vi "Intan_1dstream_to_2d_samps.vi"(8 "bytes per scan":i32=72, 9 "N data scans to read":i32=1, 10 "Nchans":i32=32, 11 "1-D  data in":u16[](array[numeric])) -> (0 "Nscans read":i32, 1 "aux_cmd_array":i32[][](array[numeric]), 2 "timestamp_array":i32[](array[numeric]), 3 "2d ADCdata_array out":u16[][](array[numeric]), 4 "Nscans underflow":bool, 5 "fragmented frame read":bool)   [LabVIEW 2015]
doc: "Reformats a 1d array of U16 Intan data (written by Teensy to serial port) into a 2-D array of data.\nThis takes Nscans worth of data, each with 36 words (= 72 bytes) worth of data, and reformats into 3 arrays:\n1. 'IN' = [73, 78] ascii values from auxiliary commands (this can be checked to verify data link)\n2. 32 bit timestamp (microseconds)\n3. Nchans (=32 for now) U16s for ADC data, with data formatted as Nchans x Nsamps\n\nRead error indicators suggest possible mis-read/mis-handling of data"
panel:
  # "2-D data output"
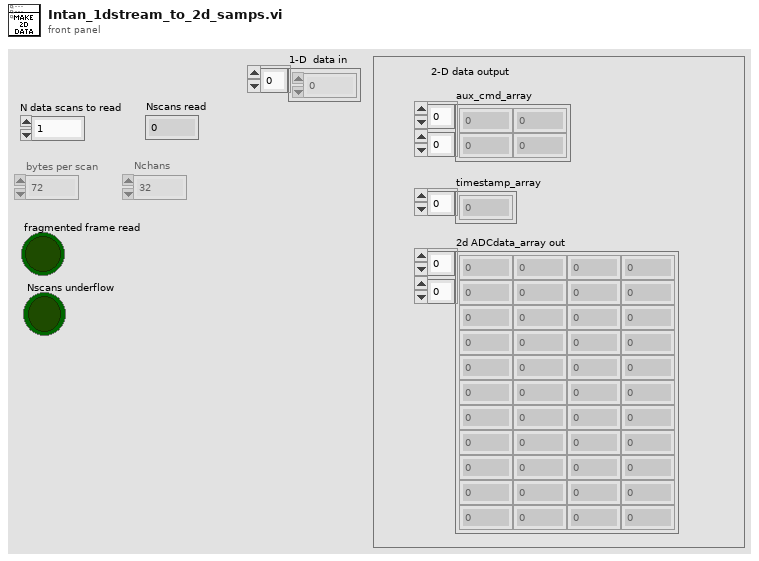
[diagram p1: front panel]
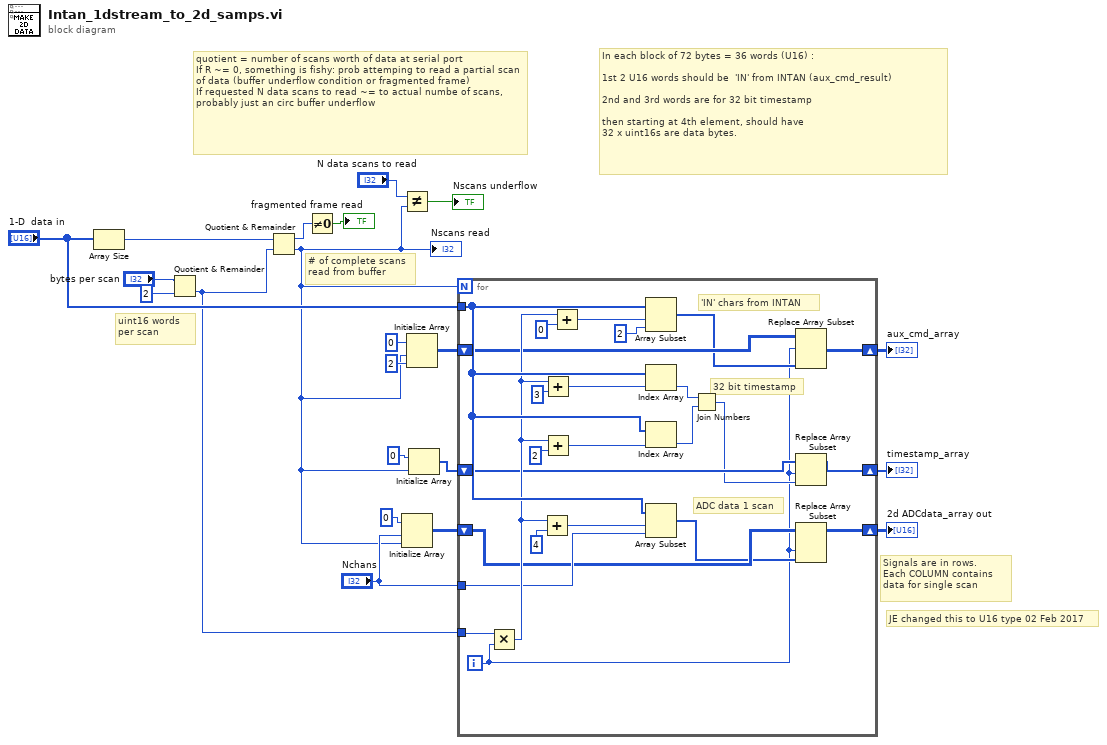
[diagram p0: block diagram]
diagram:
  # "JE changed this to U16 type 02 Feb 2017"
  # "# of complete scans\nread from buffer"
  # "Signals are in rows.\nEach COLUMN contains\ndata for single scan"
  # "In each block of 72 bytes = 36 words (U16) :\n\n1st 2 U16 words should be  'IN' from INTAN (aux_cmd_result)\n\n2nd and 3rd words are for 32 bit timestamp\n\nthen starting at 4th element, should have\n32 x uint16s are data bytes."
  # "quotient = number of scans worth of data at serial port \nIf R ~= 0, something is fishy: prob attemping to read a partial scan of data (buffer underflow condition or fragmented frame)\nIf requested N data scans to read ~= to actual numbe of scans, probably just an circ buffer underflow"
  # "uint16 words per scan"
  n1 = Array Size(array="1-D  data in") -> (size(s)=w20:i32)
  n2 = Quotient & Remainder(x="bytes per scan", y=2) -> (floor(x/y)=w15:i32)  [unwired: 1 out]
  n3 = Quotient & Remainder(x=w20, y=w15) -> (x-y*floor(x/y)=w19:i32, floor(x/y)=w1:i32)
  "Nscans read" <- w1
  n4 = Not Equal To 0?(x=w19) -> (x != 0?=→"fragmented frame read":bool)
  n5 = Not Equal?(x="N data scans to read", y=w1) -> (x != y?=→"Nscans underflow":bool)
  n6 = Initialize Array(u16 0 ("element"), "Nchans", w1) -> (w8:u16[][])
  n7 = Initialize Array(0 ("element"), w1, 2 ("dimension size")) -> (w10:i32[][])
  n8 = Initialize Array(0 ("element"), w1) -> (w9:i32[])
  n9 = for {
    N: w1 -> [_]
    tunnel: "1-D  data in" -> [w43]
    tunnel: w15 -> [w42]
    tunnel: "Nchans" -> [w32]
    shift-right: [w27] -> w3
    shift-left: w9 -> [w30]
    shift-right: [w29] -> w4
    shift-left: w10 -> [w31]
    shift-right: [w26] -> w2
    shift-left: w8 -> [w28]
    i -> [w22]
    # "ADC data 1 scan"
    # "'IN' chars from INTAN"
    # "32 bit timestamp"
    n10 = Multiply(x=w42, y=w22) -> (x*y=w40:i32)
    n11 = Add(x=w40, y=4 ("index")) -> (x+y=w33:i32)
    n12 = Add(x=w40, y=3 ("index")) -> (x+y=w35:i32)
    n13 = Add(x=w40, y=2 ("index")) -> (x+y=w34:i32)
    n14 = Add(x=w40, y=0 ("index")) -> (x+y=w36:i32)
    n15 = Array Subset(array=w43, index=w36, length=2) -> (w25:u16[])
    n16 = Index Array(array=w43, index=w35) -> (element=w45:u16)
    n17 = Index Array(array=w43, index=w34) -> (element=w44:u16)
    n18 = Array Subset(array=w43, index=w33, length=w32) -> (w23:u16[])
    n19 = Join Numbers(hi=w45, lo=w44) -> ((hi.lo)=w24:u32)
    n20 = Replace Array Subset(array=w31, new element=w25, index (row)=w22) -> (w29:i32[][])  [unwired: 1 in]
    n21 = Replace Array Subset(array=w30, new element=w24, index=w22) -> (w27:i32[])
    n22 = Replace Array Subset(array=w28, new element=w23, index (col)=w22) -> (w26:u16[][])  [unwired: 1 in]
  }
  "aux_cmd_array" <- w4
  "timestamp_array" <- w3
  "2d ADCdata_array out" <- w2
